vi "SMU_Meas_Voltage or Currentt.vi"(7 "measurement type":T1=1 caption="measurement Type" items=["Current", "Voltage"], 8 "error in (no error)":errorcluster, 10 "Channel Lists":string[](array[string]), 11 "DCPower Sessions In":refnum<k15>[](array[refnum])) -> (0 "error out":errorcluster, 2 "Measurement":dbl[][](array[numeric]), 3 "DCPower Sessions Out":refnum<k15>[](array[refnum]))   [LabVIEW 2013]
uses:
  <instrlib>/niDCPower/nidcpower.llb/niDCPower Measurement Type.ctl
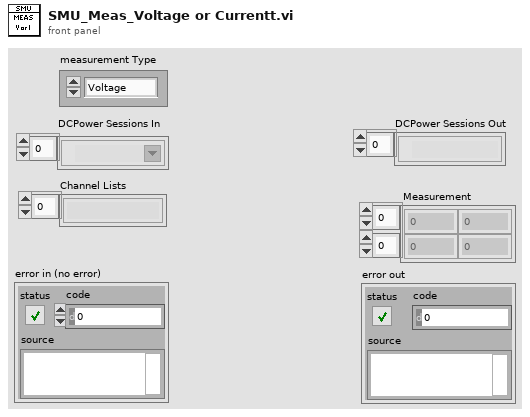
[diagram p1: front panel]
types:
  T1 = typedef "niDCPower Measurement Type.ctl" = i32
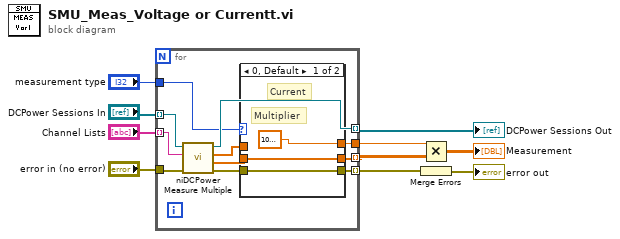
[diagram p0: block diagram]
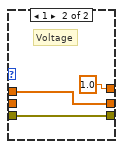
[diagram p2: hidden frame]
diagram:
  n1 = for {
    tunnel: "error in (no error)" -> [w13]
    tunnel: "DCPower Sessions In" -> [w15] mode=indexing
    tunnel: "Channel Lists" -> [w14] mode=indexing
    tunnel: [w17] -> w6 mode=indexing
    tunnel: [w21] -> w5 mode=indexing
    tunnel: [w20] -> w4 mode=indexing
    tunnel: "measurement type" -> [w12]
    tunnel: [w11] -> w1
    n2 = call <instrlib>:"niDCPower Measure Multiple.vi"("error in (no error)"=w13, "channel name"=w14, "instrument handle"=w15) -> ("error out"=w16:errorcluster, "current measurements"=w18:dbl[], "voltage measurements"=w19:dbl[], "instrument handle out"=w17:refnum<k15>)  [unwired: 5 in]
    n3 = case shown="0, Default" w12 {
      tunnel: w16 -> [w24 w26]
      tunnel: [w23 w27] -> w21
      tunnel: w19 -> [_ w27]
      tunnel: [w24 w26] -> w20
      tunnel: w18 -> [w23 _]
      tunnel: [1000000.0 1.0 ("x")] -> w11
      frame 0, Default {
        # "Multiplier"
        # "Current"
      }
      frame 1 {
        # "Voltage"
      }
    }
  }
  "DCPower Sessions Out" <- w6
  n4 = Multiply(x=w1, y=w5) -> (x*y=→"Measurement":dbl[][])
  n5 = Merge Errors(w4) -> (→"error out":errorcluster)
